vi "Series.vi"() -> ()   [LabVIEW 2009]
uses:
  Data/GetPixelData16.vi
panel:
  in  "stop":bool
  in  "count":i32
  in  "image pointers":u64[](array[numeric])
  in  "imageNo":i32 caption="Displayed image" min=0 max=10
  in  "NumImages":i32
  in  "Centre AOI":bool
  in  "AOI Width":i64
  in  "AOI Height":i64
  out "Ready":bool
  in  "Run":bool
  in  "error":errorcluster
  out "Pixel Encoding":string
  out "Intensity Graph":u16[][](graph)
  out "AOIStride":i64
  in  "PreAmp":string(combo)
  out "PixelData":u16[](array[numeric])
  out "ByteData":u8[](array[numeric])
  in  "ExposureTime":dbl
  out "ImageSizeBytes":i64
  out "Handle":i32
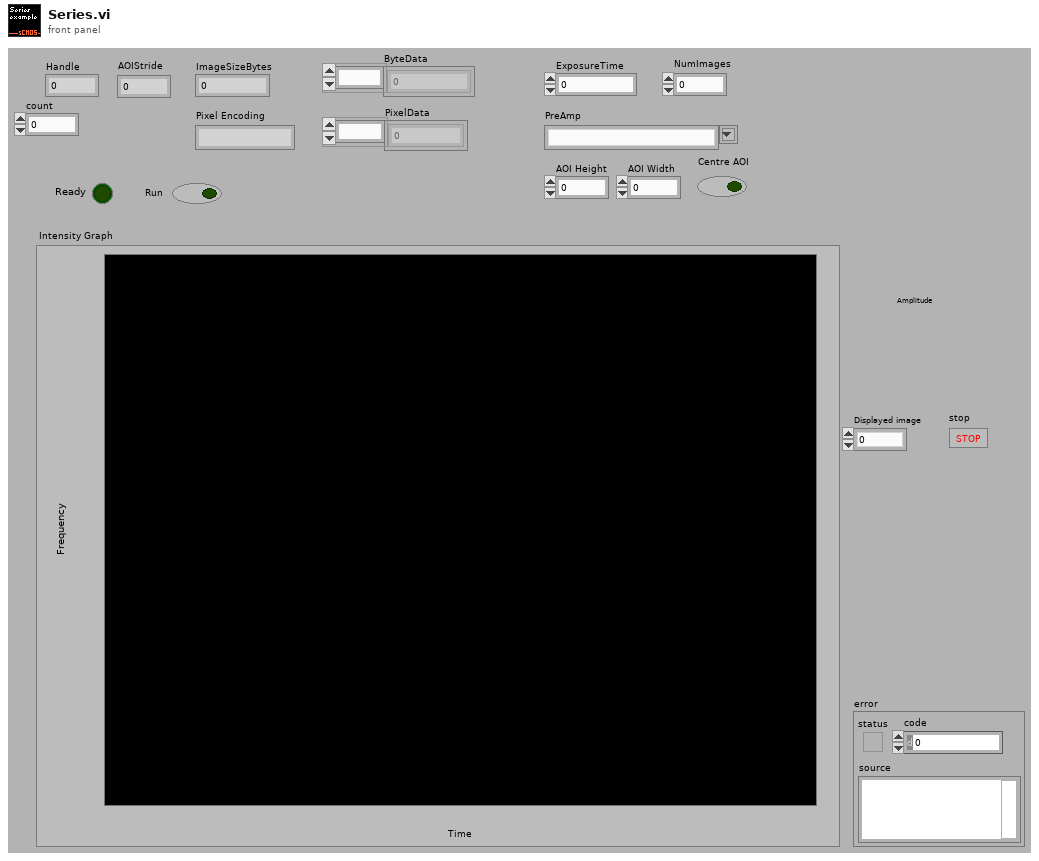
[diagram p1: front panel]
types:
  T1 = enum8{"Enabled", "Disabled", "Disabled and Grayed Out"}
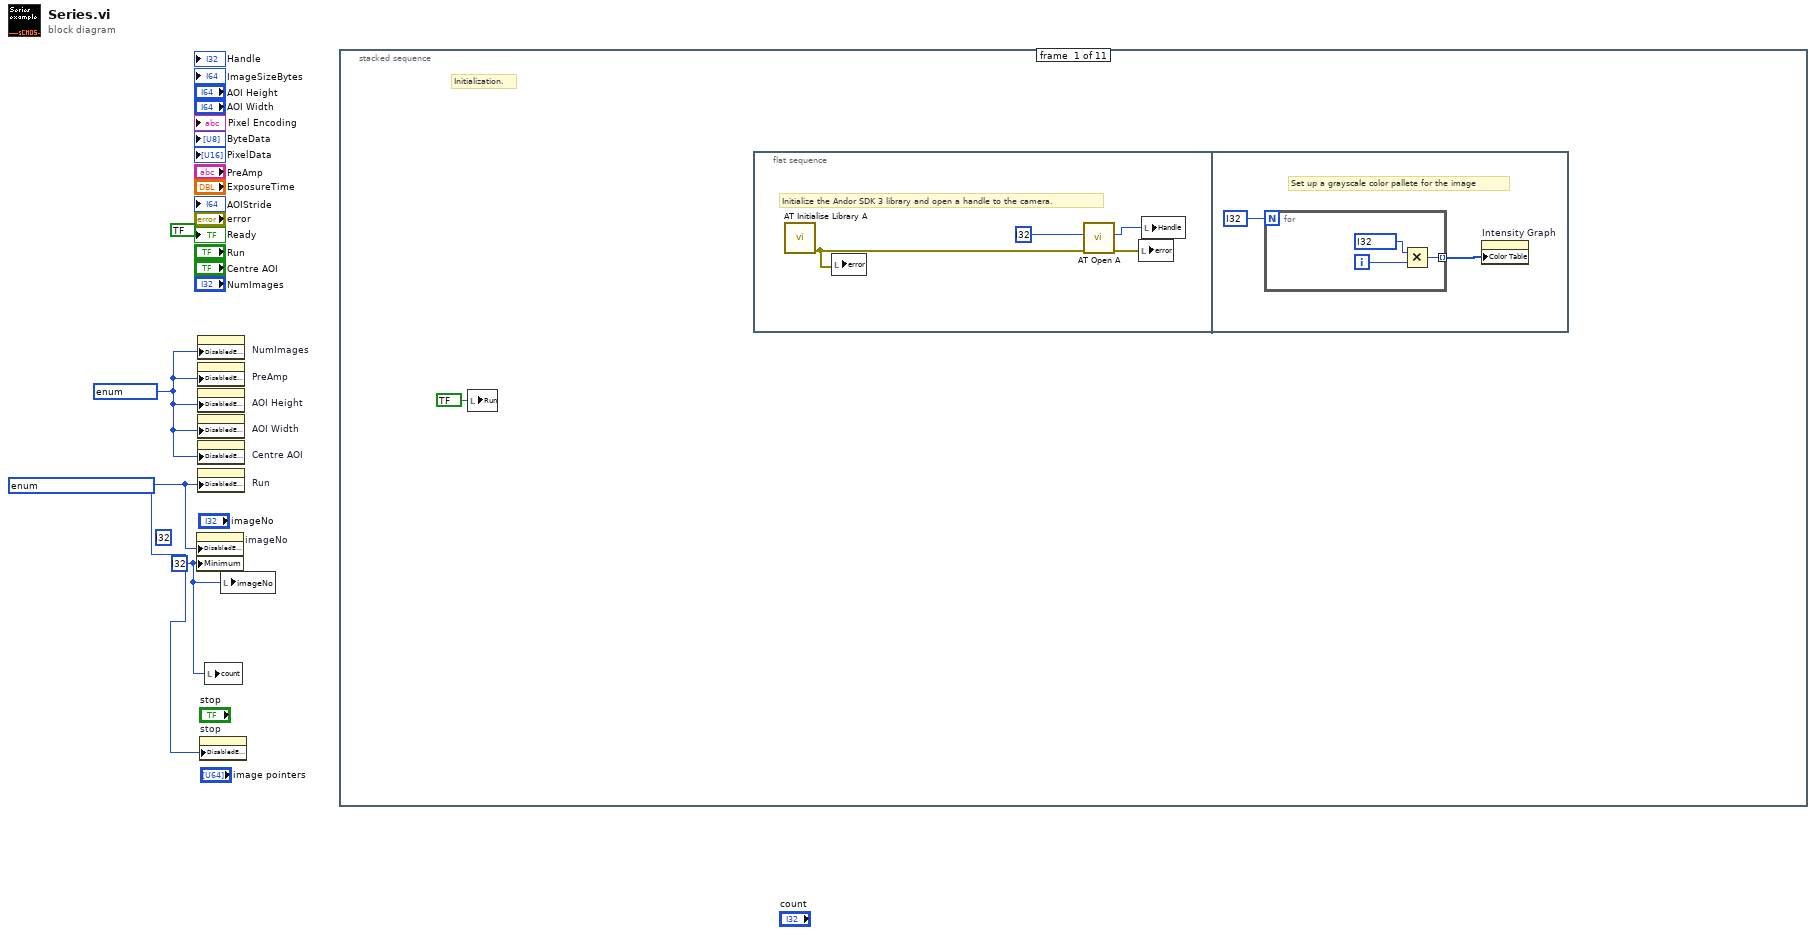
[diagram p0: block diagram]
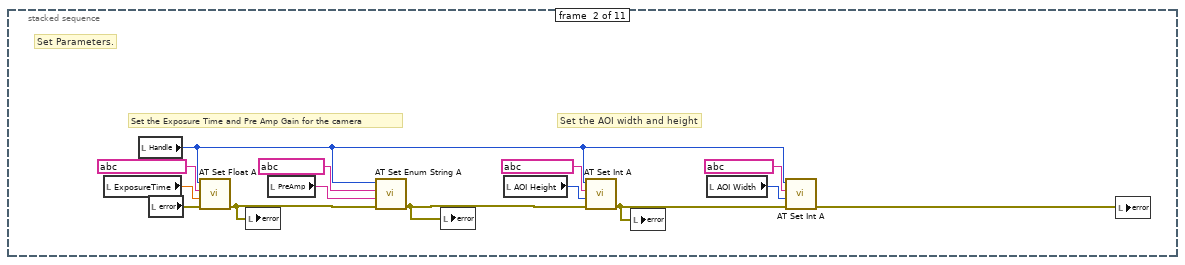
[diagram p2: hidden frame]
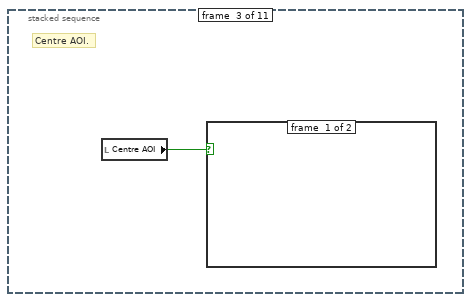
[diagram p3: hidden frame]
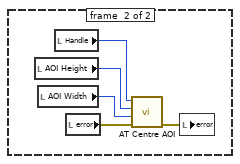
[diagram p4: hidden frame]
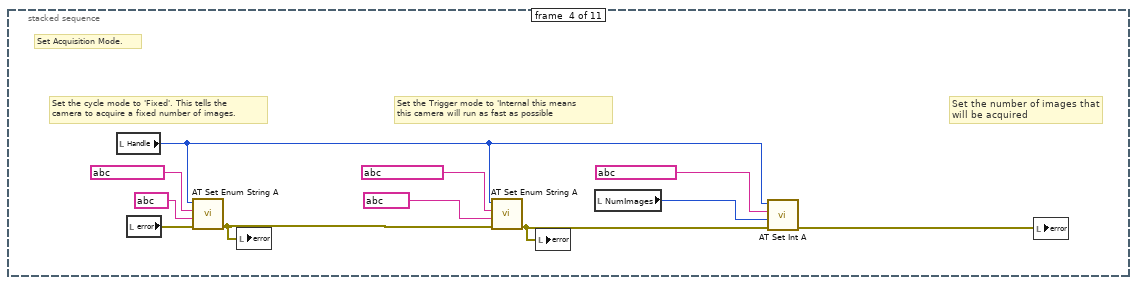
[diagram p5: hidden frame]
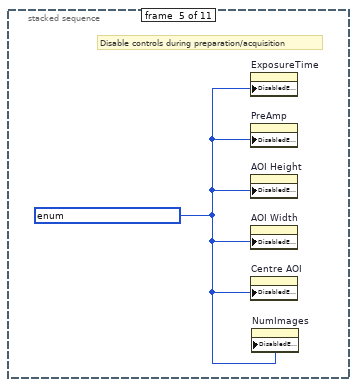
[diagram p6: hidden frame]
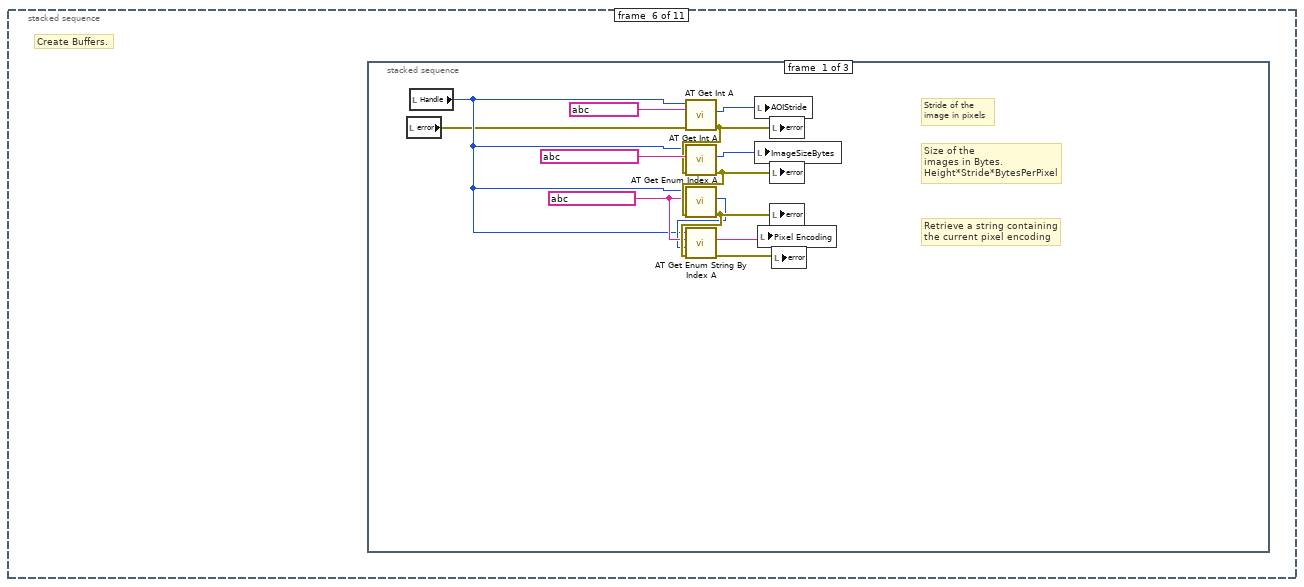
[diagram p7: hidden frame]
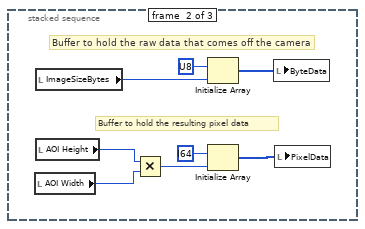
[diagram p8: hidden frame]
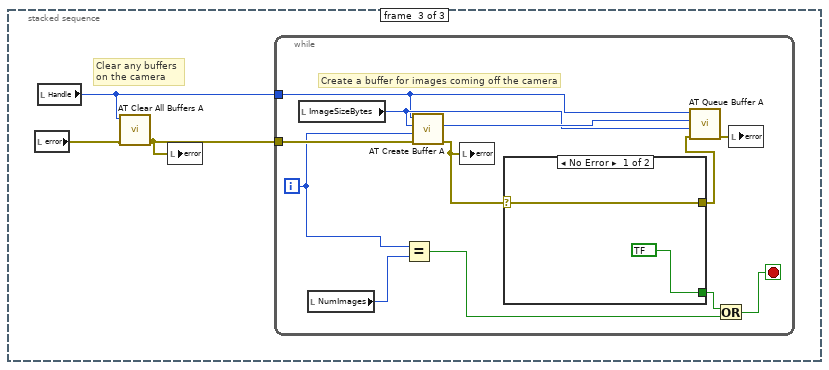
[diagram p9: hidden frame]
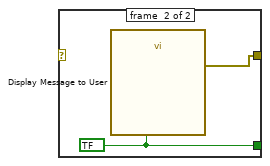
[diagram p10: hidden frame]
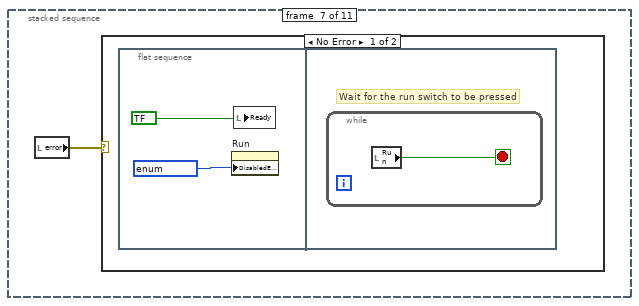
[diagram p11: hidden frame]
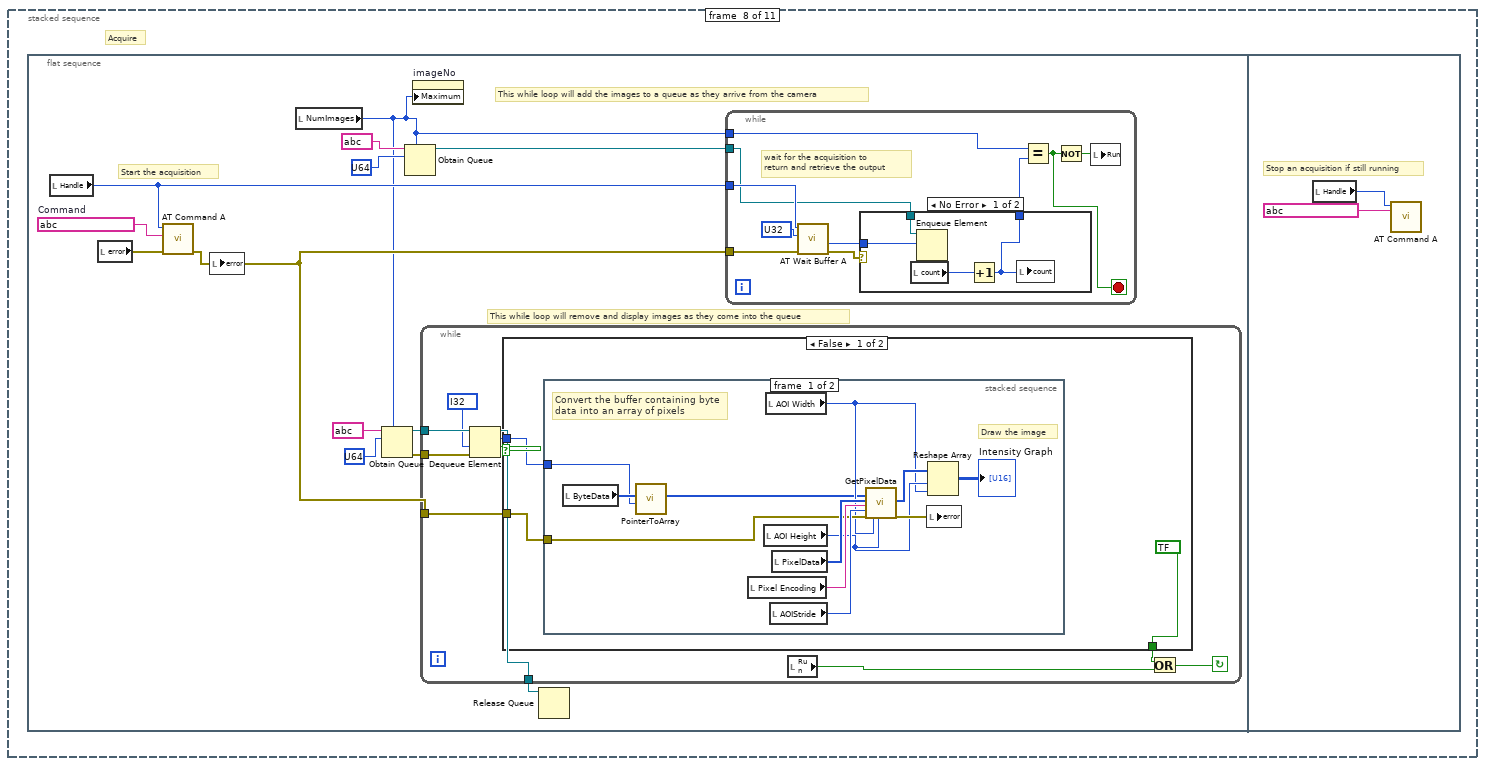
[diagram p13: hidden frame]
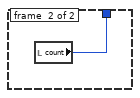
[diagram p14: hidden frame]
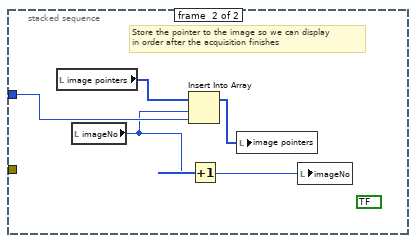
[diagram p15: hidden frame]
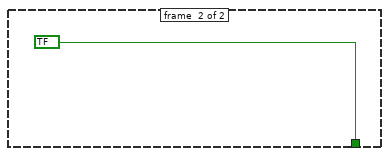
[diagram p16: hidden frame]
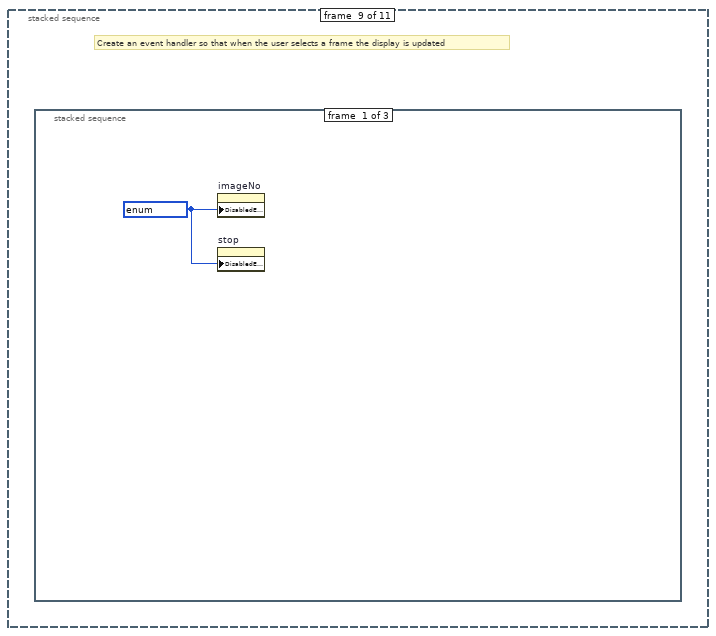
[diagram p17: hidden frame]
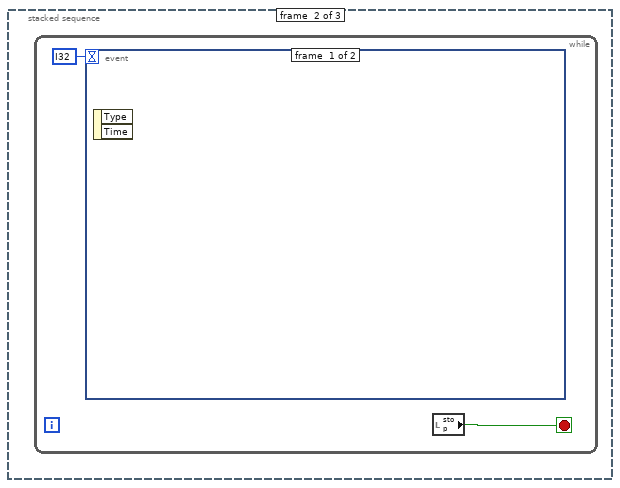
[diagram p18: hidden frame]
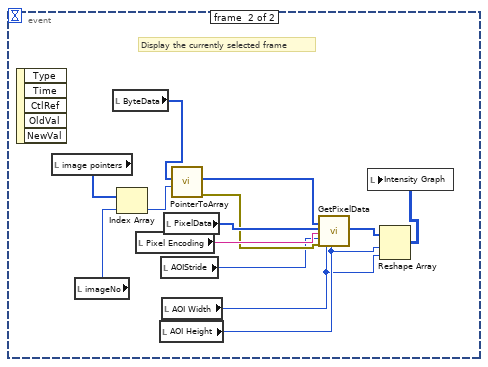
[diagram p19: hidden frame]
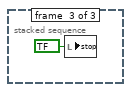
[diagram p20: hidden frame]
diagram:
  w1 = i32 ? ("Data Entry Limits:Minimum")
  (unwired) i32 ? ("Image")
  w2 = T1 ? ("Disabled")
  w3 = T1 ? ("Disabled")
  n1 = property on="imageNo" class="DigNum (strict)"("DisabledEnum"=w2, "Minimum"=w1) -> ()  [unwired: 2 in, 2 out]
  n2 = property on="NumImages" class="DigNum (strict)"("DisabledEnum"=w3) -> ()  [unwired: 2 in, 2 out]
  n3 = property on="PreAmp" class="CmbBox"("DisabledEnum"=w3) -> ()  [unwired: 2 in, 2 out]
  n4 = property on="AOI Height" class="DigNum (strict)"("DisabledEnum"=w3) -> ()  [unwired: 2 in, 2 out]
  n5 = property on="AOI Width" class="DigNum (strict)"("DisabledEnum"=w3) -> ()  [unwired: 2 in, 2 out]
  n6 = property on="Centre AOI" class="Bool (strict)"("DisabledEnum"=w3) -> ()  [unwired: 2 in, 2 out]
  n7 = property on="Run" class="Bool (strict)"("DisabledEnum"=w2) -> ()  [unwired: 2 in, 2 out]
  n8 = property on="stop" class="Bool (strict)"("DisabledEnum"=w2) -> ()  [unwired: 2 in, 2 out]
  n9 = local write "count"(w1) -> ()
  n10 = local write "imageNo"(w1) -> ()
  n11 = stacked-sequence {
    frame #0 {
      # "Initialization."
      n12 = local write "Run"(bool ? ("Run")) -> ()
      n13 = flat-sequence {
        frame #0 {
          # "Initialize the Andor SDK 3 library and open a handle to the camera."
          n14 = call "AT Initialise Library A.vi"() -> ("error out"=w7:errorcluster)  [unwired: 10 in, 1 out]
          n15 = local write "error"(w7) -> ()
          n16 = call "AT Open A.vi"("error in (no error)"=w7, "CameraIndex"=i32 ?) -> ("error out"=w6:errorcluster, "Handle"=w8:i32)  [unwired: 7 in, 1 out]
          n17 = local write "error"(w6) -> ()
          n18 = local write "Handle"(w8) -> ()
        }
        frame #1 {
          # "Set up a grayscale color pallete for the image"
          n19 = for {
            N: i32 ? -> [_]
            tunnel: [w13] -> w10 mode=indexing
            i -> [w14]
            n20 = Multiply(x=i32 ?, y=w14) -> (x*y=w13:i32)
          }
          n21 = property on="Intensity Graph" class="IntGraph (strict)"("Color Table"=w10) -> ()  [unwired: 2 in, 2 out]
        }
      }
    }
    frame #1 {
      # "Set the AOI width and height"
      # "Set the Exposure Time and Pre Amp Gain for the camera"
      # "Set Parameters."
      n22 = local read "ExposureTime"() -> (w28:dbl)
      n23 = local read "Handle"() -> (w15:i32)
      n24 = local read "error"() -> (w23:errorcluster)
      n25 = call "AT Set Float A.vi"("error in (no error)"=w23, "Value"=w28, "Feature"=string ? ("ExposureTime"), "Hndl"=w15) -> ("error out"=w26:errorcluster)  [unwired: 6 in, 1 out]
      n26 = local write "error"(w26) -> ()
      n27 = local read "PreAmp"() -> (w27:string)
      n28 = call "AT Set Enum String A.vi"("error in (no error)"=w26, "String"=w27, "Feature"=string ? ("SimplePreAmpGainControl"), "Handle"=w15) -> ("error out"=w22:errorcluster)  [unwired: 6 in, 1 out]
      n29 = local write "error"(w22) -> ()
      n30 = local read "AOI Height"() -> (w19:i64)
      n31 = call "AT Set Int A.vi"("error in (no error)"=w22, "Value"=w19, "Feature"=string ? ("Integer feature"), "Handle"=w15) -> ("error out"=w20:errorcluster)  [unwired: 6 in, 1 out]
      n32 = local write "error"(w20) -> ()
      n33 = local read "AOI Width"() -> (w18:i64)
      n34 = call "AT Set Int A.vi"("error in (no error)"=w20, "Value"=w18, "Feature"=string ? ("Integer feature 2"), "Handle"=w15) -> ("error out"=w21:errorcluster)  [unwired: 6 in, 1 out]
      n35 = local write "error"(w21) -> ()
    }
    frame #2 {
      # "Centre AOI."
      n36 = local read "Centre AOI"() -> (w29:bool)
      n37 = case shown="True" w29 {
        frame #0 {
        }
        frame #1 {
          n38 = local read "AOI Height"() -> (w31:i64)
          n39 = local read "AOI Width"() -> (w32:i64)
          n40 = local read "Handle"() -> (w30:i32)
          n41 = local read "error"() -> (w33:errorcluster)
          n42 = call "AT Centre AOI.vi"("error in (no error)"=w33, "AOI Width"=w32, "AOI Height"=w31, "Handle"=w30) -> ("error out"=w34:errorcluster)  [unwired: 7 in]
          n43 = local write "error"(w34) -> ()
        }
      }
    }
    frame #3 {
      # "Set the number of images that \nwill be acquired"
      # "Set the Trigger mode to 'Internal this means \nthis camera will run as fast as possible"
      # "Set the cycle mode to 'Fixed'. This tells the \ncamera to acquire a fixed number of images."
      # "Set Acquisition Mode."
      n44 = local read "Handle"() -> (w36:i32)
      n45 = local read "error"() -> (w43:errorcluster)
      n46 = call "AT Set Enum String A.vi"("error in (no error)"=w43, "String"=string ?, "Feature"=string ? ("Enum feature"), "Handle"=w36) -> ("error out"=w42:errorcluster)  [unwired: 6 in, 1 out]
      n47 = local write "error"(w42) -> ()
      n48 = call "AT Set Enum String A.vi"("error in (no error)"=w42, "String"=string ?, "Feature"=string ? ("Enum feature"), "Handle"=w36) -> ("error out"=w39:errorcluster)  [unwired: 6 in, 1 out]
      n49 = local write "error"(w39) -> ()
      n50 = local read "NumImages"() -> (w37:i32)
      n51 = call "AT Set Int A.vi"("error in (no error)"=w39, "Value"=w37, "Feature"=string ? ("Integer feature 2"), "Handle"=w36) -> ("error out"=w35:errorcluster)  [unwired: 6 in, 1 out]
      n52 = local write "error"(w35) -> ()
    }
    frame #4 {
      w46 = T1 ? ("Disabled")
      # "Disable controls during preparation/acquisition"
      n53 = property on="ExposureTime" class="DigNum (strict)"("DisabledEnum"=w46) -> ()  [unwired: 2 in, 2 out]
      n54 = property on="PreAmp" class="CmbBox"("DisabledEnum"=w46) -> ()  [unwired: 2 in, 2 out]
      n55 = property on="AOI Height" class="DigNum (strict)"("DisabledEnum"=w46) -> ()  [unwired: 2 in, 2 out]
      n56 = property on="AOI Width" class="DigNum (strict)"("DisabledEnum"=w46) -> ()  [unwired: 2 in, 2 out]
      n57 = property on="Centre AOI" class="Bool (strict)"("DisabledEnum"=w46) -> ()  [unwired: 2 in, 2 out]
      n58 = property on="NumImages" class="DigNum (strict)"("DisabledEnum"=w46) -> ()  [unwired: 2 in, 2 out]
    }
    frame #5 {
      # "Create Buffers."
      n59 = stacked-sequence {
        frame #0 {
          w52 = string ? ("Enum feature")
          # "Retrieve a string containing \nthe current pixel encoding"
          # "Stride of the\nimage in pixels"
          # "Size of the\nimages in Bytes.\nHeight*Stride*BytesPerPixel"
          n60 = local read "error"() -> (w47:errorcluster)
          n61 = local read "Handle"() -> (w48:i32)
          n62 = call "AT Get Int A.vi"("error in (no error)"=w47, "Feature"=string ? ("Integer feature"), "Handle"=w48) -> ("error out"=w55:errorcluster, "Value"=w59:i64)  [unwired: 6 in, 1 out]
          n63 = call "AT Get Int A.vi"("error in (no error)"=w55, "Feature"=string ? ("Integer feature"), "Handle"=w48) -> ("error out"=w54:errorcluster, "Value"=w58:i64)  [unwired: 6 in, 1 out]
          n64 = call "AT Get Enum Index A.vi"("error in (no error)"=w54, "Feature"=w52, "Handle"=w48) -> ("error out"=w53:errorcluster, "Value"=w51:i32)  [unwired: 6 in, 1 out]
          n65 = call "AT Get Enum String By Index A.vi"("error in (no error)"=w53, "Index"=w51, "Feature"=w52, "Handle"=w48) -> ("error out"=w49:errorcluster, "String"=w50:string)  [unwired: 5 in, 1 out]
          n66 = local write "AOIStride"(w59) -> ()
          n67 = local write "ImageSizeBytes"(w58) -> ()
          n68 = local write "Pixel Encoding"(w50) -> ()
          n69 = local write "error"(w55) -> ()
          n70 = local write "error"(w54) -> ()
          n71 = local write "error"(w53) -> ()
          n72 = local write "error"(w49) -> ()
        }
        frame #1 {
          # "Buffer to hold the resulting pixel data"
          # "Buffer to hold the raw data that comes off the camera"
          n73 = local read "AOI Width"() -> (w66:i64)
          n74 = local read "ImageSizeBytes"() -> (w61:i64)
          n75 = local read "AOI Height"() -> (w65:i64)
          n76 = Multiply(x=w65, y=w66) -> (x*y=w60:i64)
          n77 = Initialize Array(u8 ?, w61) -> (w63:u8[])
          n78 = Initialize Array(i64 ?, w60) -> (w64:i64[])
          n79 = local write "ByteData"(w63) -> ()
          n80 = local write "PixelData"(w64) -> ()
        }
        frame #2 {
          # "Clear any buffers \non the camera"
          n81 = local read "error"() -> (w70:errorcluster)
          n82 = local read "Handle"() -> (w68:i32)
          n83 = call "AT Clear All Buffers A.vi"("error in (no error)"=w70, "Handle"=w68) -> ("error out"=w69:errorcluster)  [unwired: 8 in, 1 out]
          n84 = local write "error"(w69) -> ()
          n85 = while {
            tunnel: w69 -> [w79]
            tunnel: w68 -> [w78]
            i -> [w74]
            stop <- w71 stop-if-true
            # "Create a buffer for images coming off the camera"
            n86 = local read "ImageSizeBytes"() -> (w81:i64)
            n87 = local read "NumImages"() -> (w75:i32)
            n88 = Equal?(x=w74, y=w75) -> (x = y?=w72:bool)
            n89 = call "AT Create Buffer A.vi"("error in (no error)"=w79, "Buffer"=w74, "Size"=w81, "Handle"=w78) -> ("error out"=w77:errorcluster, "Buffer out"=w82:u64)  [unwired: 5 in, 1 out]
            n90 = local write "error"(w77) -> ()
            n91 = case shown="No Error" w77 {
              selector: w77 -> [w84 _]
              tunnel: [w84 w86] -> w76
              tunnel: [bool ? ("Enable") w85] -> w73
              frame #0 {
              }
              frame #1 {
                w85 = bool ? ("Enable")
                n92 = call "Display Message to User"("Enable"=w85) -> ("error out"=w86:errorcluster)  [unwired: 9 in, 1 out]
              }
            }
            n93 = call "AT Queue Buffer A.vi"("error in (no error)"=w76, "PtrSize"=w81, "Ptr"=w82, "Handle"=w78) -> ("error out"=w80:errorcluster)  [unwired: 6 in, 1 out]
            n94 = Or(x=w73, y=w72) -> (x .or. y?=w71:bool)
            n95 = local write "error"(w80) -> ()
          }
        }
      }
    }
    frame #6 {
      n96 = local read "error"() -> (w87:errorcluster)
      n97 = case shown="No Error" w87 {
        frame #0 {
          n98 = flat-sequence {
            frame #0 {
              n99 = property on="Run" class="Bool (strict)"("DisabledEnum"=T1 ? ("Disabled")) -> ()  [unwired: 2 in, 2 out]
              n100 = local write "Ready"(bool ? ("Ready")) -> ()
            }
            frame #1 {
              # "Wait for the run switch to be pressed"
              n101 = while {
                stop <- w90 stop-if-true
                n102 = local read "Run"() -> (w90:bool)
              }
            }
          }
        }
        frame #1 {
        }
      }
    }
    frame #7 {
      # "Acquire"
      n103 = flat-sequence {
        frame #0 {
          w101 = string ?  # Command
          # "This while loop will remove and display images as they come into the queue"
          # "This while loop will add the images to a queue as they arrive from the camera"
          # "Start the acquisition"
          n104 = local read "Handle"() -> (w103:i32)
          n105 = local read "error"() -> (w102:errorcluster)
          n106 = call "AT Command A.vi"("error in (no error)"=w102, "Feature"=w101, "Handle"=w103) -> ("error out"=w100:errorcluster)  [unwired: 7 in, 1 out]
          n107 = local write "error"(w100) -> ()
          n108 = local read "NumImages"() -> (w91:i32)
          n109 = Obtain Queue(max queue size (-1, unlimited)=w91, name (unnamed)=string ?, element data type=u64 ?) -> (queue out=w95:refnum<queue>, error out=w96:errorcluster)  [unwired: 2 in, 1 out]
          n110 = Obtain Queue(max queue size (-1, unlimited)=w91, name (unnamed)=string ?, element data type=u64 ?) -> (queue out=w98:refnum<queue>)  [unwired: 2 in, 2 out]
          n111 = property on="imageNo" class="DigNum (strict)"("Maximum"=w91) -> ()  [unwired: 2 in, 2 out]
          n112 = while {
            tunnel: w96 -> [w128]
            tunnel: w95 -> [w127]
            tunnel: w100 -> [w126]
            tunnel: [w122] -> w92
            stop <- w121 continue-if-true
            n113 = Dequeue Element(queue=w127, timeout in ms (-1)=i32 ?, error in (no error)=w128) -> (queue out=w122:refnum<queue>, element=w124:u64, timed out?=w123:bool)  [unwired: 1 out]
            n114 = case shown="False" w123 {
              tunnel: w126 -> [w131 _]
              tunnel: w124 -> [w130 _]
              tunnel: [bool ? ("x") bool ? ("x")] -> w119
              frame #0 {
                n115 = stacked-sequence {
                  tunnel: w131 -> [w137 _]
                  tunnel: w130 -> [w132 w148]
                  frame #0 {
                    # "Draw the image"
                    # "Convert the buffer containing byte \ndata into an array of pixels"
                    n116 = local read "ByteData"() -> (w133:u8[])
                    n117 = call "PointerToArray.vi"("Pointer In"=w132, "Array in"=w133) -> ("Array out"=w134:u8[])  [unwired: 8 in, 1 out]
                    n118 = local read "Pixel Encoding"() -> (w142:string)
                    n119 = local read "AOI Height"() -> (w136:i64)
                    n120 = local read "AOI Width"() -> (w135:i64)
                    n121 = local read "AOIStride"() -> (w143:i64)
                    n122 = local read "PixelData"() -> (w141:u16[])
                    n123 = call-poly "GetPixelData.vi"("Input buffer"=w134, "Output buffer in"=w141, "Pixel Encoding"=w142, "Stride"=w143, "error in (no error)"=w137, "Width"=w135, "Height"=w136) -> ("Output buffer out"=w138:u16[], "error out"=w140:errorcluster)  [unwired: 10 in, 1 out]
                    n124 = local write "error"(w140) -> ()
                    n125 = Reshape Array(w138, w136, w135) -> (→"Intensity Graph":u16[][])
                  }
                  frame #1 {
                    (unwired) bool ? ("x")
                    # "Store the pointer to the image so we can display\nin order after the acquisition finishes"
                    n126 = local read "image pointers"() -> (w147:u64[])
                    n127 = local read "imageNo"() -> (w144:i32)
                    n128 = Insert Into Array(array=w147, index=w144, new element=w148) -> (w146:u64[])
                    n129 = Increment(x=w144) -> (x+1=w145:i32)
                    n130 = local write "image pointers"(w146) -> ()
                    n131 = local write "imageNo"(w145) -> ()
                  }
                }
              }
              frame #1 {
              }
            }
            n132 = local read "Run"() -> (w120:bool)
            n133 = Or(x=w119, y=w120) -> (x .or. y?=w121:bool)
          }
          n134 = Release Queue(queue=w92) -> ()  [unwired: 2 in, 3 out]
          n135 = while {
            tunnel: w103 -> [w112]
            tunnel: w100 -> [w111]
            tunnel: w98 -> [w110]
            tunnel: w91 -> [w106]
            stop <- w104 stop-if-true
            # "wait for the acquisition to \nreturn and retrieve the output"
            n136 = call "AT Wait Buffer A.vi"("error in (no error)"=w111, "Timeout"=u32 ?, "Handle"=w112) -> ("error out"=w107:errorcluster, "Output buffer"=w109:u64)  [unwired: 5 in, 2 out]
            n137 = case shown="No Error" w107 {
              tunnel: w110 -> [w117 _]
              tunnel: w109 -> [w116 _]
              tunnel: [w114 w118] -> w105
              frame #0 {
                n138 = local read "count"() -> (w115:i32)
                n139 = Enqueue Element(queue=w117, element=w116) -> ()  [unwired: 2 in, 3 out]
                n140 = Increment(x=w115) -> (x+1=w114:i32)
                n141 = local write "count"(w114) -> ()
              }
              frame #1 {
                n142 = local read "count"() -> (w118:i32)
              }
            }
            n143 = Equal?(x=w106, y=w105) -> (x = y?=w104:bool)
            n144 = Not(x=w104) -> (.not. x?=w108:bool)
            n145 = local write "Run"(w108) -> ()
          }
        }
        frame #1 {
          # "Stop an acquisition if still running"
          n146 = local read "Handle"() -> (w151:i32)
          n147 = call "AT Command A.vi"("Feature"=string ? ("Command"), "Handle"=w151) -> ()  [unwired: 8 in, 2 out]
        }
      }
    }
    frame #8 {
      # "Create an event handler so that when the user selects a frame the display is updated"
      n148 = stacked-sequence {
        frame #0 {
          w152 = T1 ? ("Disabled")
          n149 = property on="imageNo" class="DigNum (strict)"("DisabledEnum"=w152) -> ()  [unwired: 2 in, 2 out]
          n150 = property on="stop" class="Bool (strict)"("DisabledEnum"=w152) -> ()  [unwired: 2 in, 2 out]
        }
        frame #1 {
          n151 = while {
            stop <- w153 stop-if-true
            n152 = event shown="[1] \" imageNo\": Value Change" {
              selector: _ -> [_ _]
              dyn-events: _ -> [_ _]
              timeout: i32 ? -> [_ _]
              event #0 {
                n153 = event-data() -> ()  [unwired: 1 in, 2 out]
              }
              event #1 {
                # "Display the currently selected frame"
                n154 = event-data() -> ()  [unwired: 1 in, 5 out]
                n155 = local read "image pointers"() -> (w161:u64[])
                n156 = local read "imageNo"() -> (w155:i32)
                n157 = local read "ByteData"() -> (w166:u8[])
                n158 = Index Array(array=w161, index=w155) -> (element=w160:u64)
                n159 = local read "Pixel Encoding"() -> (w164:string)
                n160 = local read "AOI Height"() -> (w158:i64)
                n161 = local read "AOIStride"() -> (w162:i64)
                n162 = local read "AOI Width"() -> (w157:i64)
                n163 = local read "PixelData"() -> (w165:u16[])
                n164 = call "PointerToArray.vi"("Pointer In"=w160, "Array in"=w166) -> ("error out"=w163:errorcluster, "Array out"=w167:u8[])  [unwired: 8 in]
                n165 = call-poly "GetPixelData.vi"("Input buffer"=w167, "Output buffer in"=w165, "Pixel Encoding"=w164, "Stride"=w162, "error in (no error)"=w163, "Width"=w157, "Height"=w158) -> ("Output buffer out"=w159:u16[])  [unwired: 10 in, 2 out]
                n166 = Reshape Array(w159, w158, w157) -> (w156:u16[][])
                n167 = local write "Intensity Graph"(w156) -> ()
              }
            }
            n168 = local read "stop"() -> (w153:bool)
          }
        }
        frame #2 {
          n169 = local write "stop"(bool ? ("stop")) -> ()
        }
      }
    }
    frame #9 {
      w169 = T1 ? ("Disabled")
      # "re-enable controls"
      n170 = property on="AOI Height" class="DigNum (strict)"("DisabledEnum"=w169) -> ()  [unwired: 2 in, 2 out]
      n171 = property on="AOI Width" class="DigNum (strict)"("DisabledEnum"=w169) -> ()  [unwired: 2 in, 2 out]
      n172 = property on="PreAmp" class="CmbBox"("DisabledEnum"=w169) -> ()  [unwired: 2 in, 2 out]
      n173 = property on="ExposureTime" class="DigNum (strict)"("DisabledEnum"=w169) -> ()  [unwired: 2 in, 2 out]
      n174 = property on="Centre AOI" class="Bool (strict)"("DisabledEnum"=w169) -> ()  [unwired: 2 in, 2 out]
      n175 = property on="NumImages" class="DigNum (strict)"("DisabledEnum"=w169) -> ()  [unwired: 2 in, 2 out]
    }
    frame #10 {
      # "Close the current camera handle and unload the library"
      # "ShutDown."
      n176 = local write "Ready"(bool ? ("Ready")) -> ()
      n177 = local read "Handle"() -> (w171:i32)
      n178 = call "AT Clear All Buffers A.vi"("Handle"=w171) -> ("error out"=w170:errorcluster)  [unwired: 9 in, 1 out]
      n179 = call "AT Close A.vi"("error in (no error)"=w170, "Handle"=w171) -> ("error out"=w172:errorcluster)  [unwired: 8 in, 1 out]
      n180 = call "AT Finalise Library A.vi"("error in (no error)"=w172) -> ()  [unwired: 9 in, 2 out]
    }
  }
  "Ready" <- bool ? ("Ready")
